vi "EREG_PID.vi"(1 "PID gains":T1, 2 "Target Pressure (psi)":dbl, 3 "data":dynamicdata(waveform)) -> (0 "Output":dbl)   [LabVIEW 2017]
uses:
  <vilib>/addons/control/pid/pid.llb/PID (DBL).vi
  <vilib>/addons/control/pid/NI_PID_pid.lvlib
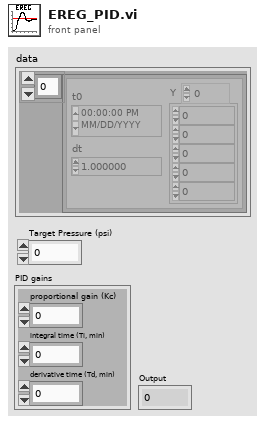
[diagram p1: front panel]
types:
  T1 = cluster{"proportional gain (Kc)":dbl, "integral time (Ti, min)":dbl, "derivative time (Td, min)":dbl}
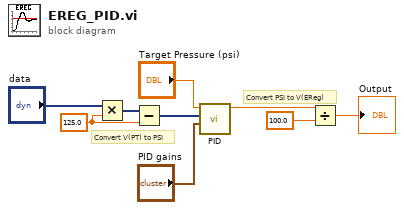
[diagram p0: block diagram]
diagram:
  w3 = 125.0 ("Multiplication factor")
  # "Convert PSI to V(EReg)"
  # "Convert V(PT) to PSI"
  n1 = Multiply(x="data", y=w3) -> (x*y=w4:dynamicdata)
  n2 = Subtract(x=w4, y=w3) -> (x-y=w7:dynamicdata)
  n3 = call-poly <vilib>:"PID.vi"("PID gains"="PID gains", "process variable"=w7, "setpoint"="Target Pressure (psi)") -> ("output"=w6:dbl)  [unwired: 7 in, 1 out]
  n4 = Divide(x=w6, y=100.0) -> (x/y=→"Output":dbl)
